vi "zdrot - Givens Rotation (CDB).vi"(5 "yInc":i32=1, 7 "xInc":i32=1, 8 "s":dbl, 9 "c":dbl=1.0, 10 "y in":cdb[](array[numeric]), 11 "x in":cdb[](array[numeric])) -> (0 "error":i32, 2 "y out":cdb[](array[numeric]), 3 "x out":cdb[](array[numeric]))   [LabVIEW 2018, in "NI_AALBLAS.lvlib"]
doc: "Applies a Givens rotation to a set of points."
uses:
  NI_AALBLAS.lvlib
  Fucntion.ctl
  BLAS1 Utility(CDB).vi
panel:
  # "x out(i)=c*x in(i)+s*y in(i)\ny out(i)=c*y in(i)-s*x in(i)"
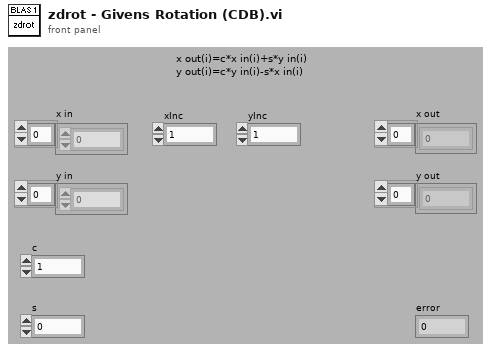
[diagram p1: front panel]
types:
  T1 = typedef "NI_AALBLAS.lvlib/Fucntion.ctl" = u16
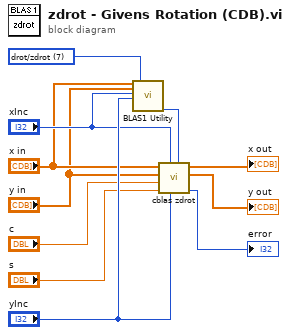
[diagram p0: block diagram]
diagram:
  w2 = T1 7 items=["ddot/zdotu/zdotc", "daxpy/zaxpy", "dnrm2/dznrm2", "dasum/dzasum", "dcopy/zcopy", "dswap/zswap", "drotm", "drot/zdrot", "idamax/izamax", "idamin/izamin", "dgemv/zgemv", "dsymv/zhemv", "dtrmv/ztrmv", "dsyr/zher", "dsyr2/zher2", "dger/zgeru/zgerc", "dtrsv/ztrsv", "dgemm/zgemm", "dsymm/zsymm/zhemm", "dtrmm/ztrmm", "dsyrk/zsyrk/zherk", "dsyr2k/zsyr2k/zher2k", "dtrsm/ztrsm"] ("function")
  n1 = call-poly "BLAS1 Utility.vi"("x"="x in", "y"="y in", "xInc"="xInc", "yInc"="yInc", "function"=w2) -> ("n"=w1:i32)  [unwired: 14 out]
  n2 = call "cblas zdrot.vi"("n"=w1, "incy"="yInc", "incx"="xInc", "s"="s", "c"="c", "y In"="y in", "x In"="x in") -> ("error"=→"error":i32, "y Out"=→"y out":cdb[], "x Out"=→"x out":cdb[])  [unwired: 2 out]
